vi "Calculate Fuel Valve Percent From RPM.vi"(11 "RPMs (double)":dbl) -> ()   [LabVIEW 2017]
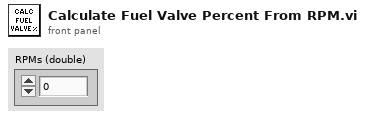
[diagram p1: front panel]
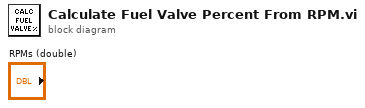
[diagram p0: block diagram]
diagram:
